vi "Serial Test.vi"(8 "error in (no error)":errorcluster, 9 "Write":bool, 10 "Command":string="*IDN?", 11 "Resource":string="FTDI") -> (0 "error out":errorcluster={"status"=TRUE, "code"=-1073807346, "source"="VISA Clear in Wrappers.lvlib:Serial.vi->Wrappers.lvlib:Serial Main.vi"}, 3 "Output":string)   [LabVIEW 2019]
uses:
  Serial/Serial.lvclass
panel:
  in  "stop":bool
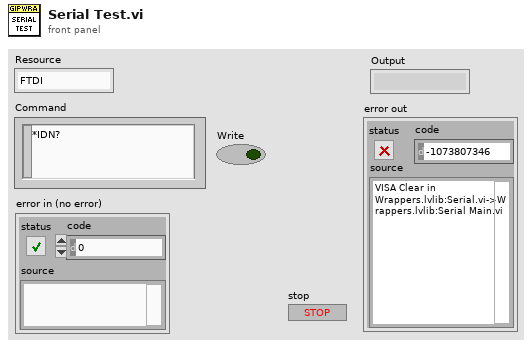
[diagram p1: front panel]
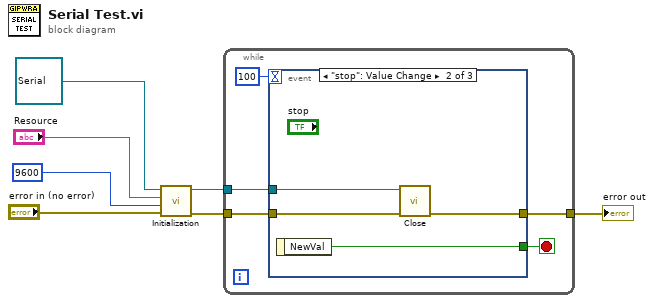
[diagram p0: block diagram]
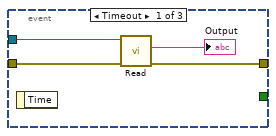
[diagram p2: hidden frame]
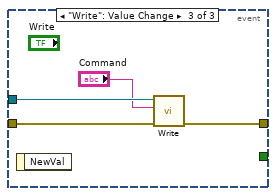
[diagram p3: hidden frame]
diagram:
  n1 = call "Initialization.vi"("error in (no error)"="error in (no error)", "baud rate"=u32 9600, "VISA Resouce"="Resource", "Serial in"=refnum<class "Serial.lvclass"> refnum ("Serial.lvclass")) -> ("error out"=w3:errorcluster, "Serial out"=w2:refnum<class "Serial.lvclass">)  [unwired: 6 in]
  n2 = while {
    tunnel: w3 -> [w11]
    tunnel: [w10] -> w7
    tunnel: w2 -> [w8]
    stop <- w12 stop-if-true
    n3 = event shown="[1] \"stop\": Value Change" {
      selector: _ -> [_ _ _]
      dyn-events: _ -> [_ _ _]
      timeout: 100 -> [_ _ _]
      tunnel: [_ w20 _] -> w12
      tunnel: [w15 w18 w22] -> w10
      tunnel: w11 -> [w16 w19 w23]
      tunnel: w8 -> [w13 w17 w24]
      event Timeout {
        n4 = event-data() -> ()  [unwired: 1 in, 1 out]
        n5 = call "Read.vi"("error in (no error)"=w16, "Serial in"=w13) -> ("error out"=w15:errorcluster, "Output"=→"Output":string)  [unwired: 7 in, 1 out]
      }
      event "stop": Value Change {
        n6 = event-data() -> ("NewVal"=w20:bool)  [unwired: 1 in]
        n7 = call "Close.vi"("error in (no error)"=w19, "Serial in"=w17) -> ("error out"=w18:errorcluster)  [unwired: 8 in, 1 out]
      }
      event "Write": Value Change {
        n8 = event-data() -> ()  [unwired: 1 in, 1 out]
        n9 = call "Write.vi"("error in (no error)"=w23, "Command"="Command", "Serial in"=w24) -> ("error out"=w22:errorcluster)  [unwired: 7 in, 1 out]
      }
    }
  }
  "error out" <- w7
